vi "Test Power Up.vi"(8 "error in (no error)":errorcluster, 11 "Application":refnum<class "Application.lvclass">) -> (0 "error out":errorcluster, 3 "result":bool)   [LabVIEW 2015, in "LCM Single-Up Power Up.lvclass"]
uses:
  LCM Single-Up Power Up.lvclass
  Classes/Application/Class/Application.lvclass
  CBTF Applications/SmartCast Testing/Main/LCM Single-Up/Application/Application/Class/typedefs/Instrument Selector -- Enum.ctl
  Classes/Instruments/USB-6001/Class/USB-6001.lvclass
  Classes/Instruments/MIO Device/Class/typedefs/Channel Type -- Enum.ctl
  Classes/Instruments/MIO Device/Class/typedefs/Read Type -- Enum.ctl
  <vilib>/Cree, Inc/Cree Test Framework/Core Launcher/Core Manager Methods -- Enum.ctl
  CBTF Applications/SmartCast Testing/Main/LCM Single-Up/Application/Application/Class/LCM Single-Up.lvclass
  Classes/Test Recipe/Class/Test Recipe.lvclass
  Classes/Instruments/MIO Device/Class/MIO Device.lvclass
  <vilib>/Cree, Inc/Cree Test Framework/Classes/Data/Data Repo/Class/Data Repo.lvclass
  <vilib>/Cree, Inc/Cree Test Framework/Core Launcher/Core Launcher.lvlib
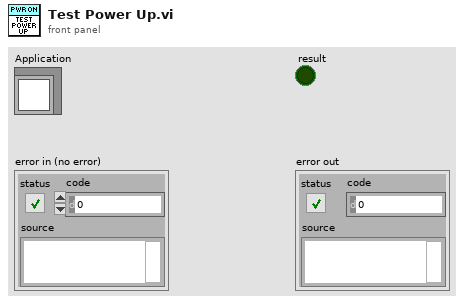
[diagram p1: front panel]
types:
  T1 = typedef "Core Launcher.lvlib/Core Manager Methods -- Enum.ctl" = enum16{"Spawn Objects", "Get Objects", "Destroy Objects"}
  T2 = typedef "MIO Device.lvlib/MIO Device.lvclass/Read Type -- Enum.ctl" = enum16{"Get All", "Get Latest", "Get Average"}
  T3 = typedef "MIO Device.lvlib/MIO Device.lvclass/Channel Type -- Enum.ctl" = enum16{"Analog Input", "Analog Output", "Digital Input", "Digital Output"}
  T4 = typedef "LCM Single-Up.lvlib/LCM Single-Up.lvclass/Instrument Selector -- Enum.ctl" = enum16{"Relay", "MIO Device", "I2C Device", "Thermocouple"}
  T5 = typedef "Application.lvlib/App Properties.lvclass/Class Properties -- Cluster.ctl" = cluster{"UUT Info":T6[], "Test Information":refnum<vi>, "Test Complete Event":refnum<user-event>, "Shop Floor System":refnum<class "Shop Floor System.lvclass">, "Gold Board":refnum<class "Golden Board.lvclass">, "Test Recipe":refnum<class "Test Recipe.lvclass">, "Instruments":refnum<class "Base Class.lvclass">[], "Mode":T7, "Test Results":cluster{"Pass":bool[], "Fail Codes":string[]}, "Station Config":refnum<class "Station Config.lvclass">}
  T6 = typedef "Application.lvlib/App Properties.lvclass/UUT Reference -- Cluster.ctl" = cluster{"Serial Number Reference":refnum<vi>, "Status Message Reference":refnum<vi>}
  T7 = typedef "Application.lvlib/Application.lvclass/Op Mode -- Enum.ctl" = u16
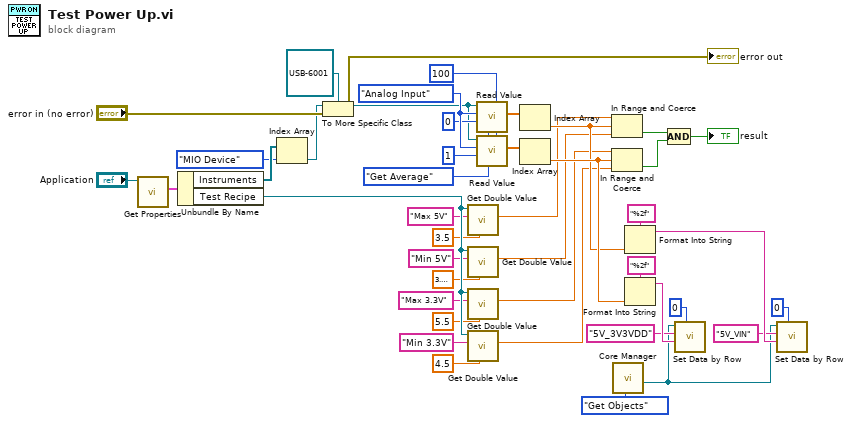
[diagram p0: block diagram]
diagram:
  w24 = Read_Type_--_Enum."Get Average" ("Read Function (Get All)")
  w23 = 100 ("Samples to Read (50)")
  w22 = Channel_Type_--_Enum."Analog Input" ("Channel Type")
  n1 = call "Get Properties.vi"("Acrobat Template in"="Application") -> ("Class Properties"=w10:T5)  [unwired: 8 in, 2 out]
  n2 = Unbundle By Name(w10) -> ("Instruments"=w8:refnum<class "Base Class.lvclass">[], "Test Recipe"=w38:refnum<class "Test Recipe.lvclass">)
  n3 = Index Array(array=w8, index=Instrument_Selector_--_Enum."MIO Device" ("Instrument")) -> (element=w6:refnum<class "Base Class.lvclass">)
  n4 = To More Specific Class(target class=refnum<class "USB-6001.lvclass"> refnum ("USB-6001"), reference=w6, error in="error in (no error)") -> (specific class reference=w1:refnum<class "USB-6001.lvclass">, error out=→"error out":errorcluster)
  n5 = call "Get Double Value.vi"("Default Value"=3.5, "Name"="Max 5V", "Test Recipe in"=w38) -> ("Value"=w39:dbl)  [unwired: 6 in, 2 out]
  n6 = call "Get Double Value.vi"("Default Value"=3.0999999999999996, "Name"="Min 5V", "Test Recipe in"=w38) -> ("Value"=w40:dbl)  [unwired: 6 in, 2 out]
  n7 = call "Get Double Value.vi"("Default Value"=5.5, "Name"="Max 3.3V", "Test Recipe in"=w38) -> ("Value"=w41:dbl)  [unwired: 6 in, 2 out]
  n8 = call "Get Double Value.vi"("Default Value"=4.5, "Name"="Min 3.3V", "Test Recipe in"=w38) -> ("Value"=w42:dbl)  [unwired: 6 in, 2 out]
  n9 = call-dynamic "Read Value.vi"("Samples to Read (50)"=w23, "Read Function (Get All)"=w24, "Channel (0)"=u32 0, "Channel Type"=w22, "Acrobat Template in"=w1) -> ("Value"=w35:dbl[])  [unwired: 4 in, 2 out]
  n10 = call-dynamic "Read Value.vi"("Samples to Read (50)"=w23, "Read Function (Get All)"=w24, "Channel (0)"=u32 1, "Channel Type"=w22, "Acrobat Template in"=w1) -> ("Value"=w36:dbl[])  [unwired: 4 in, 2 out]
  n11 = Index Array(array=w35) -> (element=w43:dbl)  [unwired: 1 in]
  n12 = Index Array(array=w36) -> (element=w44:dbl)  [unwired: 1 in]
  n13 = In Range and Coerce(upper limit=w39, x=w43, lower limit=w40) -> (In Range?=w26:bool)  [unwired: 1 out]
  n14 = In Range and Coerce(upper limit=w41, x=w44, lower limit=w42) -> (In Range?=w25:bool)  [unwired: 1 out]
  n15 = call <vilib>:"Core Manager.vi"("Method"=Core_Manager_Methods_--_Enum."Get Objects") -> ("Data Repo"=w2:refnum<class "Data Repo.lvclass">)  [unwired: 6 in, 4 out]
  n16 = Format Into String(format string="%2f", w43) -> (resulting string=w34:string)  [unwired: 2 in, 1 out]
  n17 = Format Into String(format string="%2f", w44) -> (resulting string=w31:string)  [unwired: 2 in, 1 out]
  n18 = Compound Arithmetic op=AND(w26, w25) -> (→"result":bool)
  n19 = call <vilib>:"Set Data by Row.vi"("Row"=0, "Value"=w31, "Header"="5V_3V3VDD", "Acrobat Template in"=w2) -> ()  [unwired: 6 in, 2 out]
  n20 = call <vilib>:"Set Data by Row.vi"("Row"=0, "Value"=w34, "Header"="5V_VIN", "Acrobat Template in"=w2) -> ()  [unwired: 6 in, 2 out]
